vi "Waypoint Maker.vi"(11 "GPS COM Port":refnum<visa-resource-name>) -> (3 "Instantaneous Lat, long":dbl[](array[numeric]) format="%#_9g")   [LabVIEW 2014]
panel:
  out "Corrupted Data!":bool
  in  "Stop Averaging":bool
  out "Average Lat, long":dbl[](array[numeric]) format="%#_9g"
  # "Waypoint Maker"
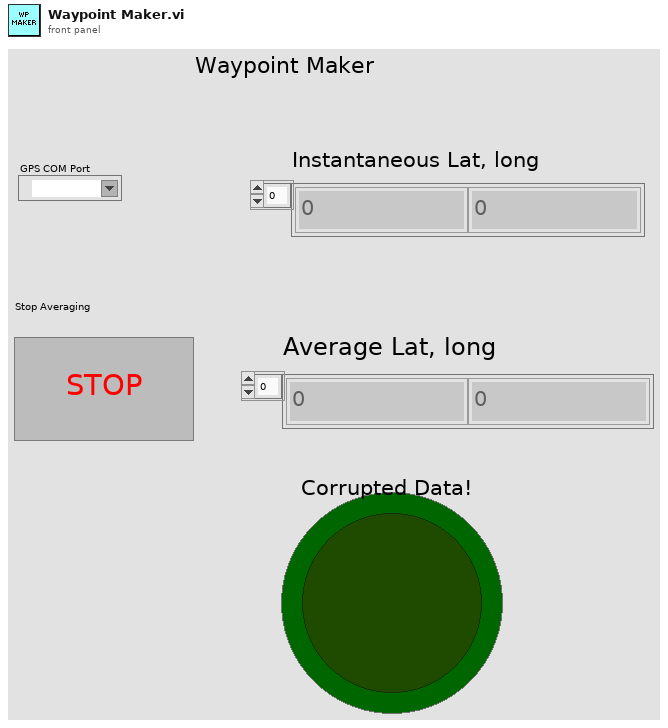
[diagram p1: front panel]
types:
  T1 = cluster{"UTC Time":timestamp, "Local Time":timestamp, "Lattitude (ddmm.mmmm)":dbl, "Lattitude North/South":string, "Longitude (ddmm.mmmm)":dbl, "Longitude East/West":string, "Magnetic Variation (degrees)":dbl, "Variation East/West":string, "Speed over ground (knots)":dbl, "Course over ground (degrees)":dbl}
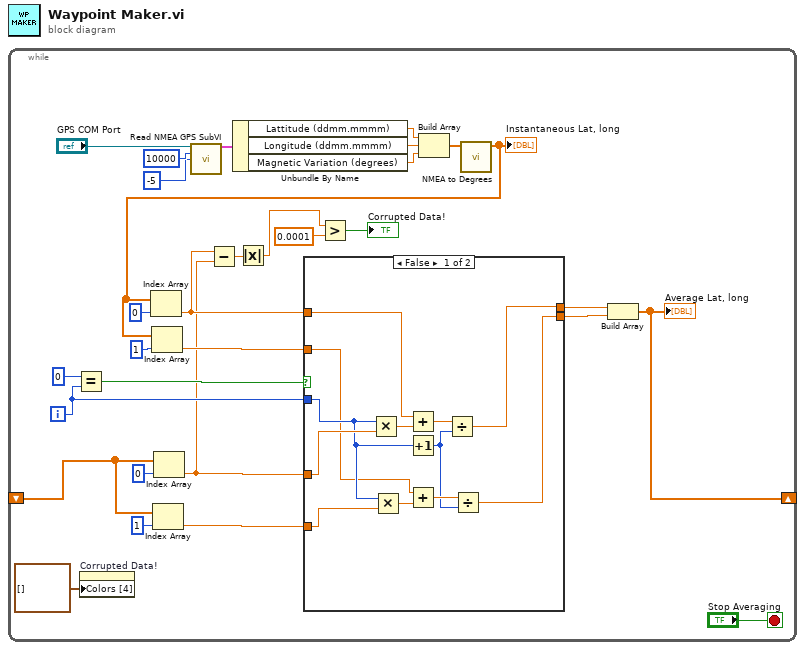
[diagram p0: block diagram]
diagram:
  n1 = while {
    shift-right: [w12] -> _
    shift-left: _ -> [w11]
    i -> [w13]
    stop <- "Stop Averaging" stop-if-true
    n2 = Equal?(x=0, y=w13) -> (x = y?=w17:bool)
    n3 = property on="Corrupted Data!" class="Bool (strict)"("Colors [4]"=cluster{u32, u32}[] []) -> ()  [unwired: 2 in, 2 out]
    n4 = Index Array(array=w11, index=1) -> (element=w8:dbl)
    n5 = Index Array(array=w11, index=0) -> (element=w5:dbl)
    n6 = call "Read NMEA GPS SubVI.vi"("VISA resource name"="GPS COM Port", "timeout (ms)"=10000, "UTC Time Zone"=-5) -> ("GPS Data"=w27:T1)  [unwired: 9 in, 3 out]
    n7 = Unbundle By Name(w27) -> ("Lattitude (ddmm.mmmm)"=w26:dbl, "Longitude (ddmm.mmmm)"=w25:dbl, "Magnetic Variation (degrees)"=w24:dbl)
    n8 = Build Array(w26, w25, w24) -> (w23:dbl[])
    n9 = call "NMEA to Degrees.vi"("NMEA Input"=w23) -> ("Degrees Output"=w21:dbl[])  [unwired: 10 in]
    "Instantaneous Lat, long" <- w21
    n10 = Index Array(array=w21, index=0) -> (element=w6:dbl)
    n11 = Index Array(array=w21, index=1) -> (element=w16:dbl)
    n12 = Subtract(x=w6, y=w5) -> (x-y=w4:dbl)
    n13 = Absolute Value(x=w4) -> (abs(x)=w2:dbl)
    n14 = case shown="False" w17 {
      tunnel: w6 -> [w40 w44]
      tunnel: w16 -> [w34 w43]
      tunnel: [w38 w44] -> w15
      tunnel: [w31 w43] -> w14
      tunnel: w13 -> [w36 _]
      tunnel: w5 -> [w42 _]
      tunnel: w8 -> [w37 _]
      frame False {
        n15 = Multiply(x=w36, y=w42) -> (x*y=w41:dbl)
        n16 = Multiply(x=w36, y=w37) -> (x*y=w35:dbl)
        n17 = Add(x=w40, y=w41) -> (x+y=w39:dbl)
        n18 = Increment(x=w36) -> (x+1=w32:i32)
        n19 = Add(x=w34, y=w35) -> (x+y=w33:dbl)
        n20 = Divide(x=w39, y=w32) -> (x/y=w38:dbl)
        n21 = Divide(x=w33, y=w32) -> (x/y=w31:dbl)
      }
      frame True {
      }
    }
    n22 = Greater?(x=w2, y=0.0001) -> (0:→"Corrupted Data!":bool)
    n23 = Build Array(w15, w14) -> (w12:dbl[])
    "Average Lat, long" <- w12
  }
